vi "SECoP_dataModifyString.vi"(7 "Position":u32, 8 "error in (no error)":errorcluster, 9 "Value":string, 10 "SECoP_dataPtr":T1 {"ptr64" format="%.0x"; "ptr32" format="%.0x"}, 11 "DLL path (in)":T2) -> (0 "error out":errorcluster, 3 "DLL path (out)":T2)   [LabVIEW 2023, in "SECoP.lvlib"]
doc: "Call <b>\"SECoP_dataModifyString.vi\"</b> to change the string value (SECoP_dataPtr).\n\n<b>DLL path</b> input and output of cluster from \"SECoP-Initialize.vi\"\n<b>SECoP_dataPtr</b> data to access\n<b>Position</b> points to a virtual flattened entry of the data type\n<b>Value</b> new value"
uses:
  SECoP.lvlib
  SECoP-libraries.ctl
  SECoP-data.ctl
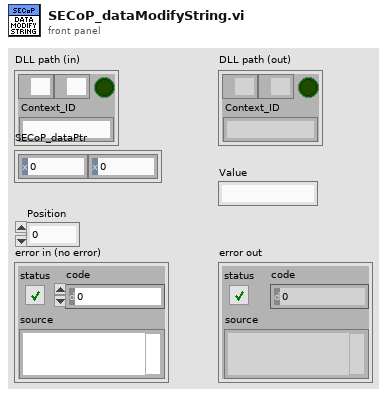
[diagram p1: front panel]
types:
  T1 = typedef "SECoP.lvlib/SECoP-data.ctl" = cluster{"ptr32":u32, "ptr64":u64}
  T2 = typedef "SECoP.lvlib/SECoP-libraries.ctl" = cluster{"serverDLL":path, "variantDLL":path, "cleanup_mode":bool, "Context_ID":string}
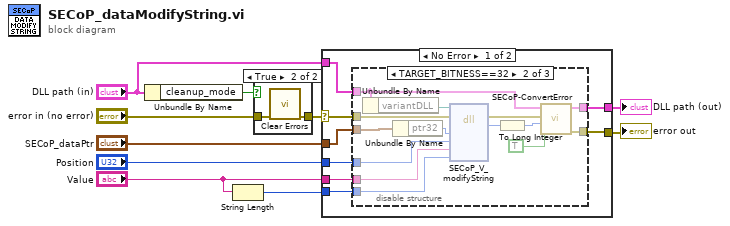
[diagram p0: block diagram]
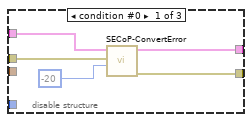
[diagram p3: hidden frame]
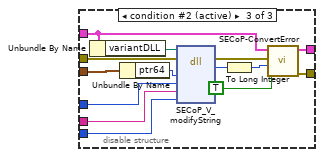
[diagram p4: hidden frame]
diagram:
  n1 = Unbundle By Name("DLL path (in)") -> ("cleanup_mode"=w8:bool)
  n2 = String Length(string="Value") -> (length=w1:i32)
  n3 = case shown="True" w8 {
    tunnel: "error in (no error)" -> [w11 w13]
    tunnel: [w11 w12] -> w6
    frame False {
    }
    frame True {
      n4 = call <vilib>:"Clear Errors.vi"("error in (no error)"=w13) -> ("error out"=w12:errorcluster)  [unwired: 5 in, 1 out]
    }
  }
  n5 = case shown="No Error" w6 {
    selector: w6 -> [w21 w55]
    tunnel: "DLL path (in)" -> [w16 w56]
    tunnel: [w18 w56] -> w10
    tunnel: [w19 w55] -> w9
    tunnel: "Position" -> [w20 _]
    tunnel: "SECoP_dataPtr" -> [w17 _]
    tunnel: "Value" -> [w15 _]
    tunnel: w1 -> [w14 _]
    frame No Error {
      n6 = disable-structure shown="TARGET_BITNESS==32" {
        disable-tunnel: w21 -> [w23 w40 w54]
        disable-tunnel: w20 -> [_ w39 w53]
        disable-tunnel: [w25 w33 w47] -> w19
        disable-tunnel: [w26 w34 w48] -> w18
        disable-tunnel: w17 -> [_ w38 w52]
        disable-tunnel: w16 -> [w24 w28 w42]
        disable-tunnel: w15 -> [_ w30 w44]
        disable-tunnel: w14 -> [_ w29 w43]
        frame condition #0 {
          n7 = call "SECoP-ConvertError.vi"("return code"=-20, "error in (no error)"=w23, "DLL path (in)"=w24) -> ("error out"=w25:errorcluster, "DLL path (out)"=w26:T2)  [unwired: 7 in]
        }
        frame condition #1 {
          n8 = Unbundle By Name(w28) -> ("variantDLL"=w27:path)
          n9 = Unbundle By Name(w38) -> ("ptr32"=w37:u32)
          n10 = dll-call lib="Z:/Praktische_Aufgaben/SECoP-LabVIEW2015/32bit/SECoP32.dll" fn="SECoP_V_modifyString"(path in=w27, error in=w40, "pData"=w37, "uPosition"=w39, "pValue"=w30, "iSize"=w29) -> (error out=w32:errorcluster, "return type"=w31:u32)  [unwired: 5 in, 1 out]
          n11 = To Long Integer(number=w31) -> (32bit integer=w35:i32)
          n12 = call "SECoP-ConvertError.vi"("return is boolean"=TRUE, "return code"=w35, "error in (no error)"=w32, "DLL path (in)"=w28) -> ("error out"=w33:errorcluster, "DLL path (out)"=w34:T2)  [unwired: 6 in]
        }
        frame condition #2 (active) {
          n13 = Unbundle By Name(w42) -> ("variantDLL"=w41:path)
          n14 = Unbundle By Name(w52) -> ("ptr64"=w51:u64)
          n15 = dll-call lib="Z:/Praktische_Aufgaben/SECoP-LabVIEW2015/32bit/SECoP32.dll" fn="SECoP_V_modifyString"(path in=w41, error in=w54, "pData"=w51, "uPosition"=w53, "pValue"=w44, "iSize"=w43) -> (error out=w46:errorcluster, "return type"=w45:u32)  [unwired: 5 in, 1 out]
          n16 = To Long Integer(number=w45) -> (32bit integer=w49:i32)
          n17 = call "SECoP-ConvertError.vi"("return is boolean"=TRUE, "return code"=w49, "error in (no error)"=w46, "DLL path (in)"=w42) -> ("error out"=w47:errorcluster, "DLL path (out)"=w48:T2)  [unwired: 6 in]
        }
      }
    }
    frame Error {
    }
  }
  "DLL path (out)" <- w10
  "error out" <- w9
